vi "Thread@Thread Jump__Parameter.vi"(1 "ParamterIn":string) -> (0 "ParamterOut":string)   [LabVIEW 2020]
uses:
  MainFrame/Global.vi
panel:
  in  "Logic":string(combo)
  in  "Thread Label":string(combo)
  in  "Confirm":bool
  # "Thread@Thread Jump $Label(,$Logic)"
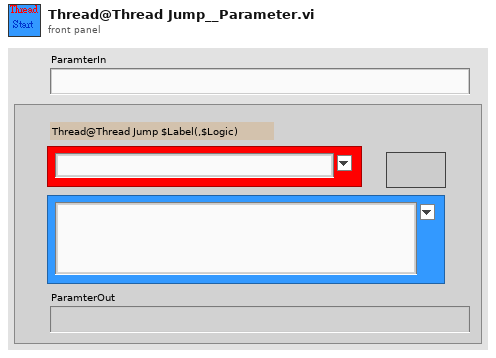
[diagram p1: front panel]
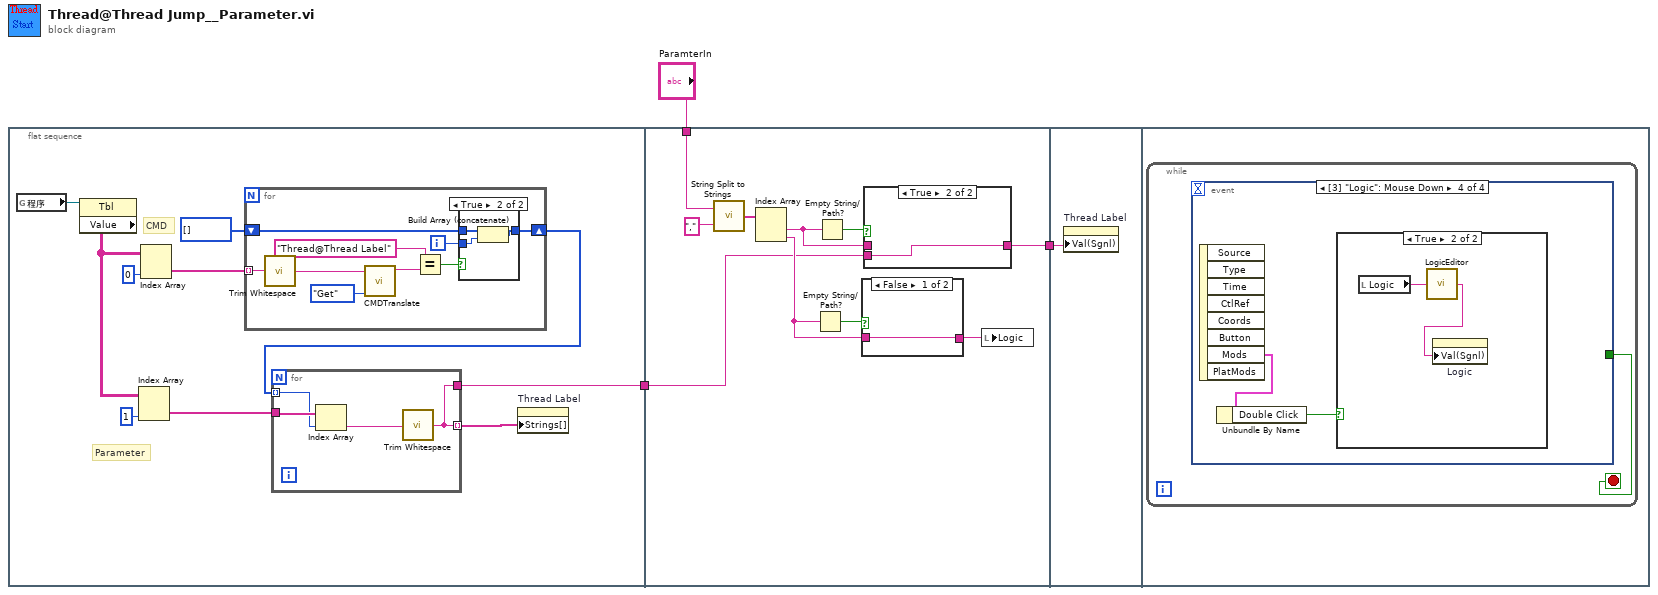
[diagram p0: block diagram]
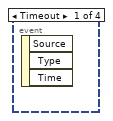
[diagram p5: hidden frame]
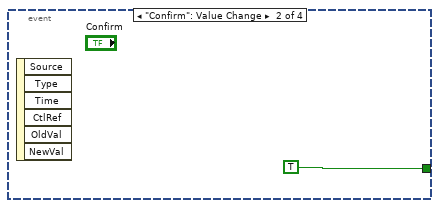
[diagram p6: hidden frame]
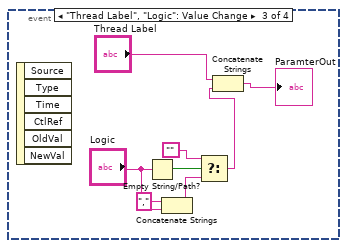
[diagram p7: hidden frame]
diagram:
  n1 = flat-sequence {
    tunnel: [w4] -> w1
    tunnel: "ParamterIn" -> [w38]
    tunnel: [w33] -> w2
    tunnel: w1 -> [w31]
    tunnel: w2 -> [w44]
    frame #0 {
      # "Parameter"
      # "CMD"
      n2 = global read "Global.vi" "程序"() -> (w13:refnum<vi>)
      n3 = property class="Tbl"(reference=w13) -> ("Value"=w10:string[][])  [unwired: 1 in, 2 out]
      n4 = Index Array(array=w10, index (col)=1 ("index (row)")) -> (element=w7:string[])  [unwired: 1 in]
      n5 = Index Array(array=w10, index (col)=0 ("index (row)")) -> (element=w9:string[])  [unwired: 1 in]
      n6 = for {
        tunnel: w9 -> [w19] mode=indexing
        shift-right: [w21] -> w6
        shift-left: i32[] [] -> [w23]
        i -> [w22]
        n7 = call <vilib>:"Trim Whitespace.vi"("string"=w19) -> ("trimmed string"=w18:string)  [unwired: 1 in]
        n8 = call "CMDTranslate.vi"("OP"=enum16{"Init", "Set", "Get", "GetInverse"}."Get", "CMDIn"=w18) -> ("CMDOut"=w20:string)  [unwired: 9 in]
        n9 = Equal?(x="Thread@Thread Label", y=w20) -> (x = y?=w24:bool)
        n10 = case shown="True" w24 {
          tunnel: w23 -> [w27 w30]
          tunnel: w22 -> [_ w29]
          tunnel: [w27 w28] -> w21
          frame False {
          }
          frame True {
            n11 = Build Array (concatenate)(w30, w29) -> (w28:i32[])
          }
        }
      }
      n12 = for {
        tunnel: w7 -> [w17]
        tunnel: w6 -> [w16] mode=indexing
        tunnel: [w15] -> w5 mode=indexing
        tunnel: [w15] -> w4
        n13 = Index Array(array=w17, index=w16) -> (element=w14:string)
        n14 = call <vilib>:"Trim Whitespace.vi"("string"=w14) -> ("trimmed string"=w15:string)  [unwired: 1 in]
      }
      n15 = property on="Thread Label" class="CmbBox"("Strings[]"=w5) -> ()  [unwired: 2 in, 2 out]
    }
    frame #1 {
      n16 = call "String Split to Strings.vi"("search string/char (-)"=",", "String"=w38) -> ("Array"=w40:string[])
      n17 = Index Array(array=w40) -> (element #1=w36:string, element #2=w34:string)  [unwired: 2 in]
      n18 = Empty String/Path?(string/path=w34) -> (empty?=w35:bool)
      n19 = Empty String/Path?(string/path=w36) -> (empty?=w37:bool)
      n20 = case shown="False" w35 {
        tunnel: w34 -> [w41 _]
        tunnel: [w41 _] -> w32
        frame False {
        }
        frame True {
        }
      }
      n21 = case shown="True" w37 {
        tunnel: w36 -> [w42 _]
        tunnel: [w42 w43] -> w33
        tunnel: w31 -> [_ w43]
        frame False {
        }
        frame True {
        }
      }
      n22 = local write "Logic"(w32) -> ()
    }
    frame #2 {
      n23 = property on="Thread Label" class="CmbBox"("Val(Sgnl)"=w44) -> ()  [unwired: 2 in, 2 out]
    }
    frame #3 {
      n24 = while {
        stop <- w45 stop-if-true
        n25 = event shown="[3] \"Logic\": Mouse Down" {
          selector: _ -> [_ _ _ _]
          dyn-events: _ -> [_ _ _ _]
          timeout: _ -> [_ _ _ _]
          tunnel: [_ TRUE _ _] -> w45
          event Timeout {
            n26 = event-data() -> ()  [unwired: 1 in, 3 out]
          }
          event "Confirm": Value Change {
            n27 = event-data() -> ()  [unwired: 1 in, 6 out]
          }
          event "Thread Label", "Logic": Value Change {
            n28 = event-data() -> ()  [unwired: 1 in, 6 out]
            n29 = Empty String/Path?(string/path="Logic") -> (empty?=w53:bool)
            n30 = Concatenate Strings("," ("string"), "Logic") -> (w51:string)
            n31 = Select(t="", s=w53, f=w51) -> (s? t:f=w48:string)
            n32 = Concatenate Strings("Thread Label", w48) -> (→"ParamterOut":string)
          }
          event "Logic": Mouse Down {
            n33 = event-data() -> ("Mods"=w56:cluster{"Double Click":bool, "Menu Key":bool})  [unwired: 1 in, 7 out]
            n34 = Unbundle By Name(w56) -> ("Double Click"=w55:bool)
            n35 = case shown="True" w55 {
              frame False {
              }
              frame True {
                n36 = local read "Logic"() -> (w58:string)
                n37 = call "LogicEditor.vi"("Logic Express"=w58) -> ("LogicExpressOut"=w57:string)
                n38 = property on="Logic" class="CmbBox"("Val(Sgnl)"=w57) -> ()  [unwired: 2 in, 2 out]
              }
            }
          }
        }
      }
    }
  }
